vi "Execute.vi"(0 "reference in":refnum<class "GetCurrentInfoCommand.lvclass">, 11 "Error In":errorcluster) -> (4 "reference out":refnum<class "GetCurrentInfoCommand.lvclass">, 15 "Error Out":errorcluster)   [LabVIEW 2024, in "GetCurrentInfoCommand.lvclass"]
doc: "Updates MediaPlayer Current Information cluster"
uses:
  GetCurrentInfoCommand.lvclass
  Receiver/MediaPlayer_class/MediaPlayer.lvclass
  GetCurrentInfoCommand.lvclass/GetCurrentInfoCommand.ctl
panel:
  # "Connector Pane"
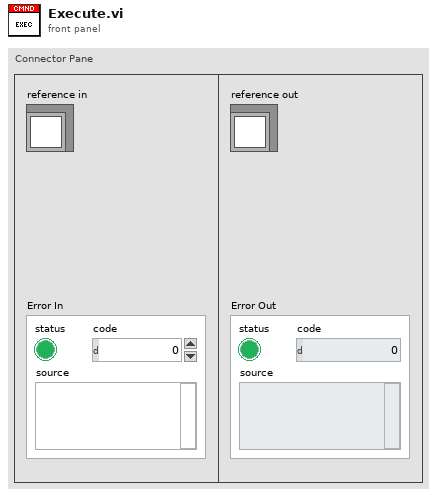
[diagram p1: front panel]
types:
  T1 = typedef "GetCurrentInfoCommand.lvclass/ObjectAttributes.ctl" = cluster{"MediaPlayerRef":refnum<class "MediaPlayer.lvclass">}
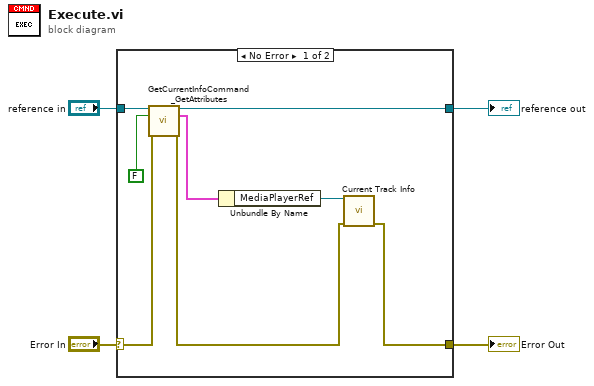
[diagram p0: block diagram]
diagram:
  n1 = case shown="No Error" "Error In" {
    selector: "Error In" -> [w12 w14]
    tunnel: [w6 w14] -> w3
    tunnel: [w9 w13] -> w1
    tunnel: "reference in" -> [w10 w13]
    frame No Error {
      n2 = call "GetCurrentInfoCommand_GetAttributes.vi"("reference in"=w10, "OnlyGetDvrReference(False)"=FALSE, "Error In"=w12) -> ("reference out"=w9:refnum<class "GetCurrentInfoCommand.lvclass">, "Data"=w11:T1, "Error Out"=w7:errorcluster)  [unwired: 9 in, 1 out]
      n3 = Unbundle By Name(w11) -> ("MediaPlayerRef"=w8:refnum<class "MediaPlayer.lvclass">)
      n4 = call-dynamic "Current Track Info.vi"("reference in"=w8, "Error In"=w7) -> ("Error Out"=w6:errorcluster)  [unwired: 12 in, 1 out]
    }
    frame Error {
    }
  }
  "Error Out" <- w3
  "reference out" <- w1
